vi "RSZVB Get Display Line.vi"(8 "error in (no error)":errorcluster {"code" format="%.0x"}, 10 "Channel (Trace) (1)":i32=1, 11 "VISA session":refnum<visa-resource-name>) -> (0 "error out":errorcluster {"code" format="%.0x"}, 1 "Display Line":bool, 2 "Position":dbl format="%^.3e", 3 "dup VISA session":refnum<visa-resource-name>)   [LabVIEW 2011]
doc: "This VI returns if the display line associated to the active trace in a Cartesian diagram area is active or not and returns its position.\n\nRemote-control command(s):\nCALCulate<Ch/Tr>:DLINe:STATe?\nCALCulate<Ch/Tr>:DLINe?"
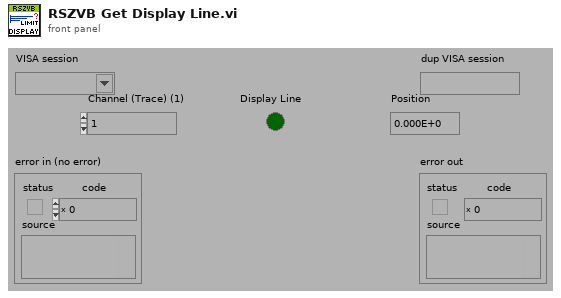
[diagram p1: front panel]
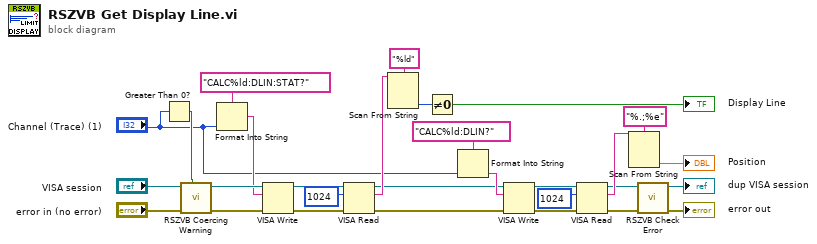
[diagram p0: block diagram]
diagram:
  n1 = Greater Than 0?(x="Channel (Trace) (1)") -> (x > 0?=w15:bool)
  n2 = call "RSZVB Coercing Warning.vi"("In Range?"=w15, "error in (no error)"="error in (no error)", "VISA session"="VISA session") -> ("error out"=w23:errorcluster, "dup VISA session"=w24:refnum<visa-resource-name>)  [unwired: 7 in]
  n3 = Format Into String(format string="CALC%ld:DLIN:STAT?", "Channel (Trace) (1)") -> (resulting string=w22:string)  [unwired: 2 in, 1 out]
  n4 = VISA Write(VISA resource name=w24, write buffer=w22, error in (no error)=w23) -> (VISA resource name out=w20:refnum<visa-resource-name>, error out=w21:errorcluster)  [unwired: 1 out]
  n5 = VISA Read(VISA resource name=w20, byte count=u32 1024 ("byte count (0)"), error in (no error)=w21) -> (VISA resource name out=w4:refnum<visa-resource-name>, read buffer=w27:string, error out=w5:errorcluster)  [unwired: 1 out]
  n6 = Scan From String(format string="%ld", input string=w27) -> (output 1=w26:i32)  [unwired: 3 in, 3 out]
  n7 = Not Equal To 0?(x=w26) -> (x != 0?=→"Display Line":bool)
  n8 = Format Into String(format string="CALC%ld:DLIN?", "Channel (Trace) (1)") -> (resulting string=w12:string)  [unwired: 2 in, 1 out]
  n9 = VISA Write(VISA resource name=w4, write buffer=w12, error in (no error)=w5) -> (VISA resource name out=w14:refnum<visa-resource-name>, error out=w13:errorcluster)  [unwired: 1 out]
  n10 = VISA Read(VISA resource name=w14, byte count=u32 1024 ("byte count (0)"), error in (no error)=w13) -> (VISA resource name out=w2:refnum<visa-resource-name>, read buffer=w11:string, error out=w3:errorcluster)  [unwired: 1 out]
  n11 = Scan From String(format string="%.;%e", input string=w11) -> (output 1=→"Position":dbl)  [unwired: 3 in, 3 out]
  n12 = call "RSZVB Check Error.vi"("error in (no error)"=w3, "VISA session"=w2) -> ("error out"=→"error out":errorcluster, "dup VISA session"=→"dup VISA session":refnum<visa-resource-name>)  [unwired: 8 in]
